vi "Points Difference.vi"(1 "# of Points (Consumer Loop)":i32, 2 "Points Missed Control Refnuma":refnum<vi>, 3 "# of Points (Producer Loop)":i32) -> (0 "Points Missed":i32)   [LabVIEW 2010]
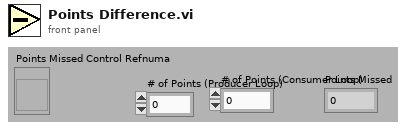
[diagram p1: front panel]
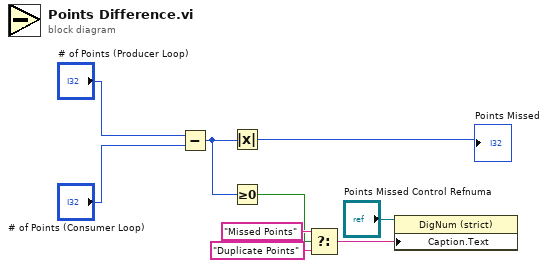
[diagram p0: block diagram]
diagram:
  n1 = Subtract(x="# of Points (Producer Loop)", y="# of Points (Consumer Loop)") -> (x-y=w8:i32)
  n2 = Absolute Value(x=w8) -> (abs(x)=→"Points Missed":i32)
  n3 = Greater Or Equal To 0?(x=w8) -> (x >= 0?=w4:bool)
  n4 = Select(t="Missed Points", s=w4, f="Duplicate Points") -> (s? t:f=w7:string)
  n5 = property on="Property Node" class="DigNum (strict)"(reference="Points Missed Control Refnuma", "Caption.Text"=w7) -> ()  [unwired: 1 in, 2 out]
